vi "DiscardBead.vi"(10 "ResultManager":T1, 11 "Bead index":i32) -> ()   [LabVIEW 2011]
uses:
  qtrk/QTrk.llb/ResultManagerInstance.ctl
  Typedefs/CmdEnum_UserInterfaceCmd.ctl
  GlobalVariables.vi
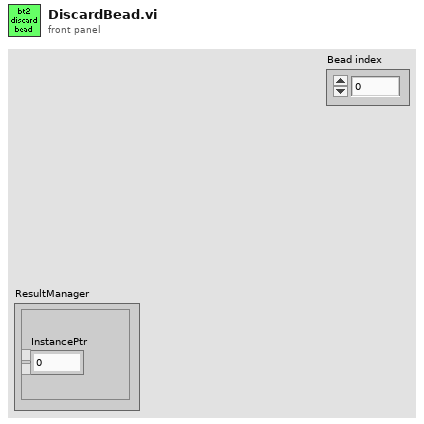
[diagram p1: front panel]
types:
  T1 = typedef "ResultManagerInstance.ctl" = cluster{"InstancePtr":u64}
  T2 = typedef "CmdEnum_UserInterfaceCmd.ctl" = enum32{"Idle (Use for default)", "ResultTracesUpdated", "MeasureConfigUpdated", "MeasureEnd", "MeasureStart"}
  T3 = typedef "MeasureConfigType.ctl" = cluster{"Bead locations":cluster{"X":i32, "Y":i32}[], "ROI":i32, "Experiment base path":path, "Image output subdir":string, "Output mode":T4, "Traces output subdir":string, "QTrk Settings":T5, "Tracking Config":T6, "Experiment Name":string, "Program":T9, "ZLUT":sgl[][][], "Camera settings":T16, "Experiment Script":string, "Max frames in memory":i32, "Save traces as binary":bool, "Pixel Calibration Gain Image":string, "Pixel Calibration Offset Image":string, "Use pixel calibration images":bool, "Internal camera settings":string}
  T4 = typedef "MeasureConfigOutputMode.ctl" = enum16{"None", "Track", "SaveImages"}
  T5 = typedef "QTrkSettings.ctl" = cluster{"Image width":i32, "Image height":i32, "Number of threads (CPU based)":i32, "CUDA Device":i32, "COM Background correction factor":sgl, "ZLUT MinRadius":sgl, "ZLUT Radial sample density":sgl, "ZLUT Angular sample density":sgl, "ZLUT ROI Coverage":sgl, "QI Iterations":i32, "QI MinRadius":sgl, "QI Radial sample density":sgl, "QI Angular sample density":sgl, "QI ROI Coverage":sgl, "QI Angular Step \nIteration Factor":sgl, "XCOR Profile Length":i32, "XCOR Profile Width":i32, "XCOR Iterations":i32, "Gaussian 2D Fit Iterations":i32, "Gaussian 2D Sigma (pixels)":sgl}
  T6 = typedef "TrackingConfigType.ctl" = cluster{"Number of steps":i32, "ZLUT stepsize (um)":sgl, "Z correction factor":sgl, "Start piezo Z (um)":sgl, "Pixel size (nm)":sgl, "2D Localization Type":T7, "Z Command (None)":T8, "Z Piezo scale":bool}
  T7 = typedef "QTrkLocalizationType.ctl" = enum16{"Center-of-Mass", "1D Cross-Correlation", "Quadrant Interpolation", "Gaussian 2D MLE", "QI + ZLUTAlign", "ZLUTAlign"}
  T8 = typedef "QTrkZCommandType.ctl" = enum16{"Nothing", "ComputeZ", "BuildRadialZLUT", "BuildImageZLUT", "RadialZLUT+ImageZLUT"}
  T9 = typedef "ExperimentProgramType.ctl" = cluster{"Commands":T10[], "Motor Axis accuracy conditions":T13, "Axis flags":T15}
  T10 = typedef "ExProgCommandType.ctl" = cluster{"cmd":T11, "axis":T12, "value/pos":dbl, "speed":dbl, "name":string}
  T11 = typedef "ExProgCommandEnumType.ctl" = enum16{"wait", "move", "acquire", "idle", "rmove", "when", "section", "stop"}
  T12 = typedef "MotorAxisEnum.ctl" = enum16{"no axis", "magrot", "magpos", "px", "py", "pz", "camx", "camy"}
  T13 = typedef "MotorPosType.ctl" = cluster{"Magnet Z":dbl, "Magnet rotation":dbl, "Camera":T14, "Piezo XY":T14, "Piezo Z":dbl}
  T14 = typedef "XYf.ctl" = cluster{"X":sgl, "Y":sgl}
  T15 = typedef "MotorPosFlagsType.ctl" = cluster{"Magnet Z":bool, "Magnet rotation":bool, "Camera":cluster{"X":bool, "Y":bool}, "Piezo XY":cluster{"X":bool, "Y":bool}, "Piezo Z":bool}
  T16 = typedef "GenericCameraConfigType.ctl" = cluster{"Framerate (Hz)":i32, "Exposure time (us)":i32, "Image size":cluster{"Width":i32, "Height":i32}, "Number of buffers":i32}
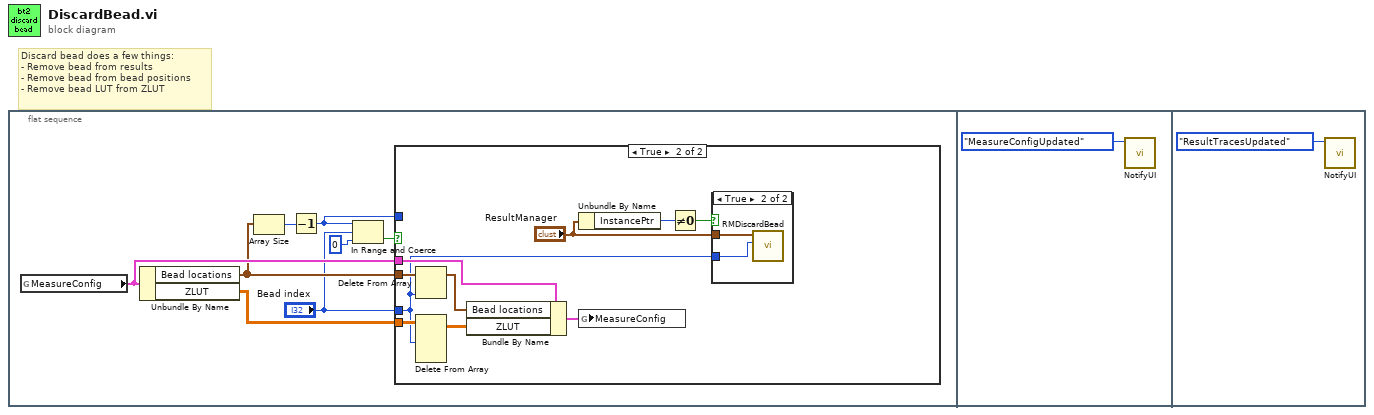
[diagram p0: block diagram]
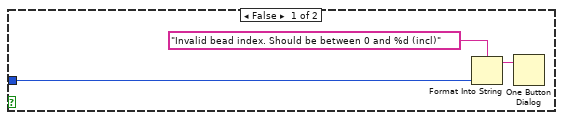
[diagram p2: hidden frame]
diagram:
  # "Discard bead does a few things:\n- Remove bead from results\n- Remove bead from bead positions\n- Remove bead LUT from ZLUT"
  n1 = flat-sequence {
    frame #0 {
      n2 = global read "GlobalVariables.vi" "MeasureConfig"() -> (w8:T3)
      n3 = Unbundle By Name(w8) -> ("Bead locations"=w6:cluster{"X":i32, "Y":i32}[], "ZLUT"=w7:sgl[][][])
      n4 = Array Size(array=w6) -> (size(s)=w2:i32)
      n5 = Decrement(x=w2) -> (x-1=w1:i32)
      n6 = In Range and Coerce(upper limit=w1, x="Bead index", lower limit=0) -> (In Range?=w3:bool)  [unwired: 1 out]
      n7 = case shown="True" w3 {
        tunnel: w8 -> [_ w21]
        tunnel: w7 -> [_ w18]
        tunnel: w6 -> [_ w16]
        tunnel: "Bead index" -> [_ w12]
        tunnel: w1 -> [w11 _]
        frame False {
          n8 = Format Into String(format string="Invalid bead index. Should be between 0 and %d (incl)" ("message"), w11) -> (resulting string=w10:string)  [unwired: 2 in, 1 out]
          n9 = One Button Dialog(message=w10) -> ()  [unwired: 1 in, 1 out]
        }
        frame True {
          n10 = Delete From Array(array=w16, index=w12) -> (array with subset deleted=w20:cluster{"X":i32, "Y":i32}[])  [unwired: 1 in, 1 out]
          n11 = Delete From Array(array=w18, index (dim 0)=w12) -> (array with subset deleted=w17:sgl[][][])  [unwired: 3 in, 1 out]
          n12 = Bundle By Name(cluster=w21, "Bead locations"=w20, "ZLUT"=w17) -> (w19:T3)
          n13 = Unbundle By Name("ResultManager") -> ("InstancePtr"=w15:u64)
          n14 = global write "GlobalVariables.vi" "MeasureConfig"(w19) -> ()
          n15 = Not Equal To 0?(x=w15) -> (x != 0?=w14:bool)
          n16 = case shown="True" w14 {
            tunnel: "ResultManager" -> [_ w23]
            tunnel: w12 -> [_ w22]
            frame False {
            }
            frame True {
              n17 = call "RMDiscardBead.vi"("beadIndex"=w22, "ResultManager"=w23) -> ()  [unwired: 9 in, 1 out]
            }
          }
        }
      }
    }
    frame #1 {
      n18 = call "NotifyUI.vi"("User Interface Commands"=CmdEnum_UserInterfaceCmd."MeasureConfigUpdated") -> ()  [unwired: 11 in]
    }
    frame #2 {
      n19 = call "NotifyUI.vi"("User Interface Commands"=CmdEnum_UserInterfaceCmd."ResultTracesUpdated") -> ()  [unwired: 11 in]
    }
  }
